vi "Get String Variable.vi"(7 "Path":string, 8 "error in (no error)":errorcluster, 9 "Default Value":string, 11 "JSON Variable in":refnum<class "JSON Variable.lvclass">) -> (0 "error out":errorcluster, 1 "Data":string, 3 "JSON Variable out":refnum<class "JSON Variable.lvclass">)   [LabVIEW 2019, in "JSON Variable.lvclass"]
uses:
  JSON Variable.lvclass
  8b948938-97d9-4327-9428-58b3f509b3f5.vi
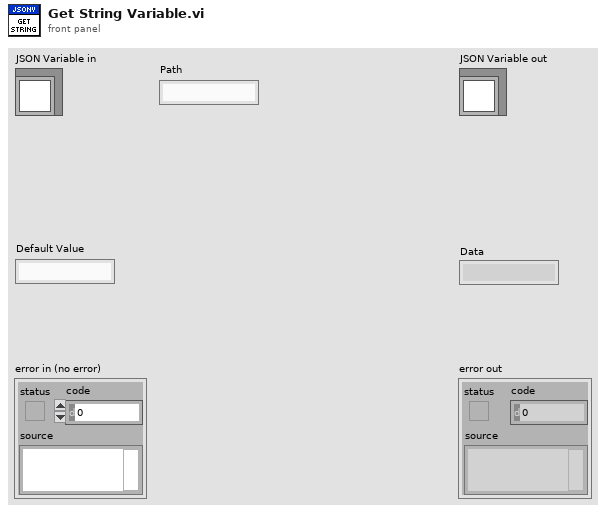
[diagram p1: front panel]
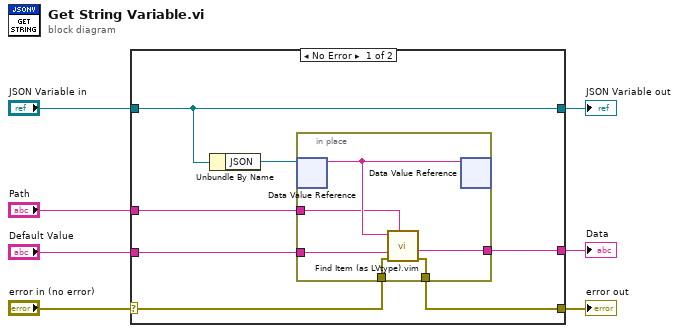
[diagram p0: block diagram]
diagram:
  n1 = case shown="No Error" "error in (no error)" {
    selector: "error in (no error)" -> [w10 w22]
    tunnel: [w9 w22] -> w6
    tunnel: [w14 w21] -> w4
    tunnel: "JSON Variable in" -> [w14 w21]
    tunnel: "Path" -> [w12 _]
    tunnel: "Default Value" -> [w11 _]
    tunnel: [w8 _] -> w1
    frame No Error {
      n2 = Unbundle By Name(w14) -> ("JSON"=w13:refnum<data-value>)
      n3 = in-place {
        in-place-border: w12 -> [w19]
        in-place-border: w11 -> [w18]
        in-place-border: w10 -> [w17]
        in-place-border: [w16] -> w9
        in-place-border: [w15] -> w8
        n4 = in-place-dvr #1(w13) -> (w20:string)  [unwired: 1 out]
        n5 = call "Find Item (as LVtype).vim"("$Path or Item Name"=w19, "error in (no error)"=w17, "Data Type and Default Value"=w18, "JSON"=w20) -> ("error out"=w16:errorcluster, "Data"=w15:string)  [unwired: 4 in, 2 out]
        n6 = in-place-dvr #1(w20) -> ()  [unwired: 2 out]
      }
    }
    frame Error {
    }
  }
  "error out" <- w6
  "JSON Variable out" <- w4
  "Data" <- w1
